vi "数组的基本使用.vi"() -> ()   [LabVIEW 2018]
panel:
  out "第3列":dbl[](array[numeric])
  out "第3行第3行":dbl[](array[numeric])
  out "第3行 第4列":dbl
  out "第2行 第3列":dbl
  out "大小":i32[](array[numeric])
  out "数组 5":dbl[][](array[numeric])
  out "数组 3":dbl[][](array[numeric])
  out "布尔":bool
  out "数组":bool[](array[boolean])
  out "数组 2":dbl[](array[numeric])
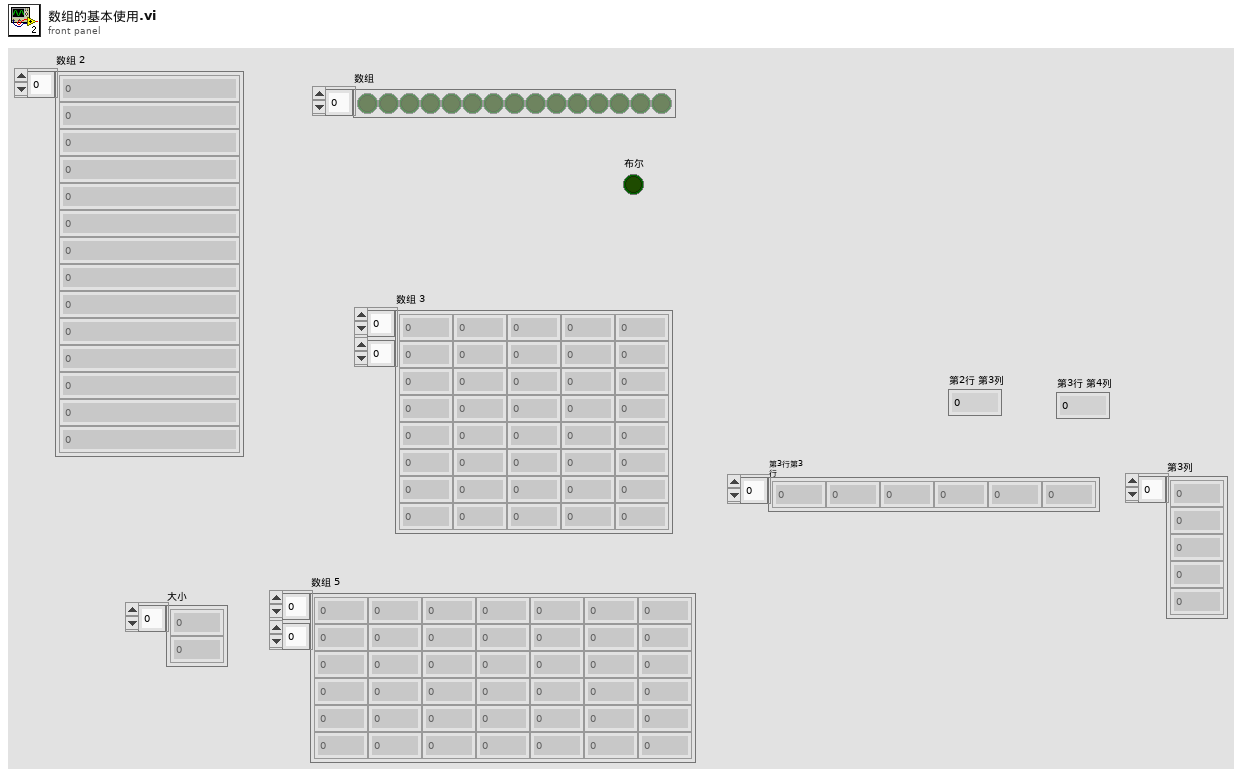
[diagram p1: front panel]
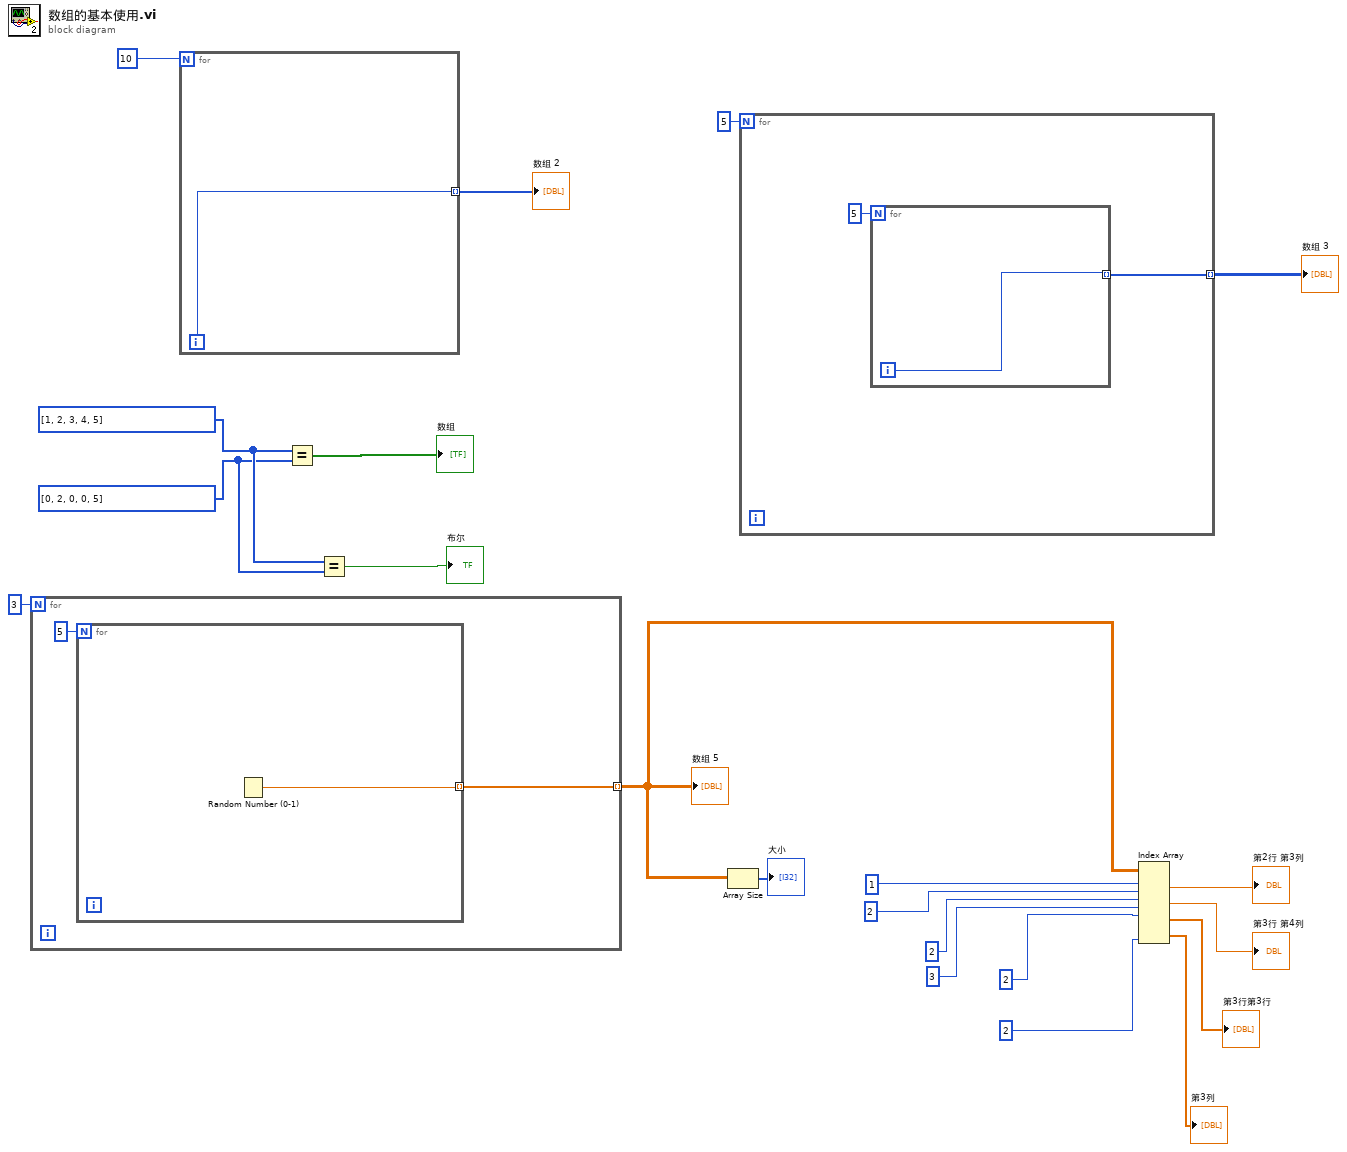
[diagram p0: block diagram]
diagram:
  w17 = i32[] [0, 2, 0, 0, 5]
  w18 = i32[] [1, 2, 3, 4, 5]
  n1 = for {
    N: 3 -> [_]
    tunnel: [w22] -> w10 mode=indexing
    n2 = for {
      N: 5 -> [_]
      tunnel: [w24] -> w22 mode=indexing
      n3 = Random Number (0-1)() -> (number: 0 to 1=w24:dbl)
    }
  }
  "数组 5" <- w10
  n4 = for {
    N: 10 -> [_]
    tunnel: [w25] -> w20 mode=indexing
    i -> [w25]
  }
  "数组 2" <- w20
  n5 = Equal?(x=w18, y=w17) -> (x = y?=→"数组":bool[])
  n6 = Equal?(x=w18, y=w17) -> (x = y?=→"布尔":bool)
  n7 = Array Size(array=w10) -> (size(s)=→"大小":i32[])
  n8 = for {
    N: 5 -> [_]
    tunnel: [w26] -> w14 mode=indexing
    n9 = for {
      N: 5 -> [_]
      tunnel: [w28] -> w26 mode=indexing
      i -> [w28]
    }
  }
  "数组 3" <- w14
  n10 = Index Array(array=w10, index (row) #1=1, index (col) #1=2, index (row) #2=2, index (col) #2=3, index (row) #3=2, index (col) #4=2) -> (element #1=→"第2行 第3列":dbl, element #2=→"第3行 第4列":dbl, element #3=→"第3行第3行":dbl[], element #4=→"第3列":dbl[])  [unwired: 2 in]
